vi "Start Drive Ref.vi"(8 "error in":errorcluster, 9 "Variant":variant, 10 "cluster":T2 {"Gyro"."Sample Rate" min=0.25 max=100.0 step=0.25}, 11 "VI in":T1) -> (0 "error out":errorcluster)   [LabVIEW 2016, in "Drive System.lvlib"]
uses:
  Drive System.lvlib
  <vilib>/Rock Robotics/WPI/Solenoid/WPI_SolenoidChannel.ctl
  <vilib>/Rock Robotics/WPI/Solenoid/WPI_SolenoidDevRef.ctl
  Varient Cmd Types/Lock Command.ctl
  <vilib>/Rock Robotics/SystemInterfaces/spilib/spi_bus.ctl
  <vilib>/Rock Robotics/SystemInterfaces/AI/FPGA_AIChannel.ctl
  <vilib>/Rock Robotics/WPI/Gyro/WPI_GyroDevRef.ctl
  <vilib>/Rock Robotics/SystemInterfaces/Encoder/FPGA_EncoderIdx.ctl
  <vilib>/Rock Robotics/WPI/Encoder/WPI_EncoderType.ctl
  <vilib>/Rock Robotics/SystemInterfaces/Counter/FPGA_CounterCtrSystemIndex.ctl
  <vilib>/Rock Robotics/WPI/Encoder/WPI_EncoderDevRef.ctl
  <vilib>/Rock Robotics/SystemInterfaces/DIO/FPGA_DIOPWMChannel.ctl
  <vilib>/Rock Robotics/WPI/PWM/WPI_PWMDeadband.ctl
  <vilib>/Rock Robotics/WPI/MotorControl/WPI_MotorControlType.ctl
  <vilib>/Rock Robotics/WPI/MotorControl/WPI_MotorControlDeviceRef.ctl
  <vilib>/Rock Robotics/WPI/RobotDrive/WPI_RobotDriveDevRef.ctl
  DriveCmdList.ctl
  DriveCmd.ctl
  DriveMainType.ctl
  Drive Refs/Drive Ref Type.ctl
panel:
  # "Analog"
  # "XRS"
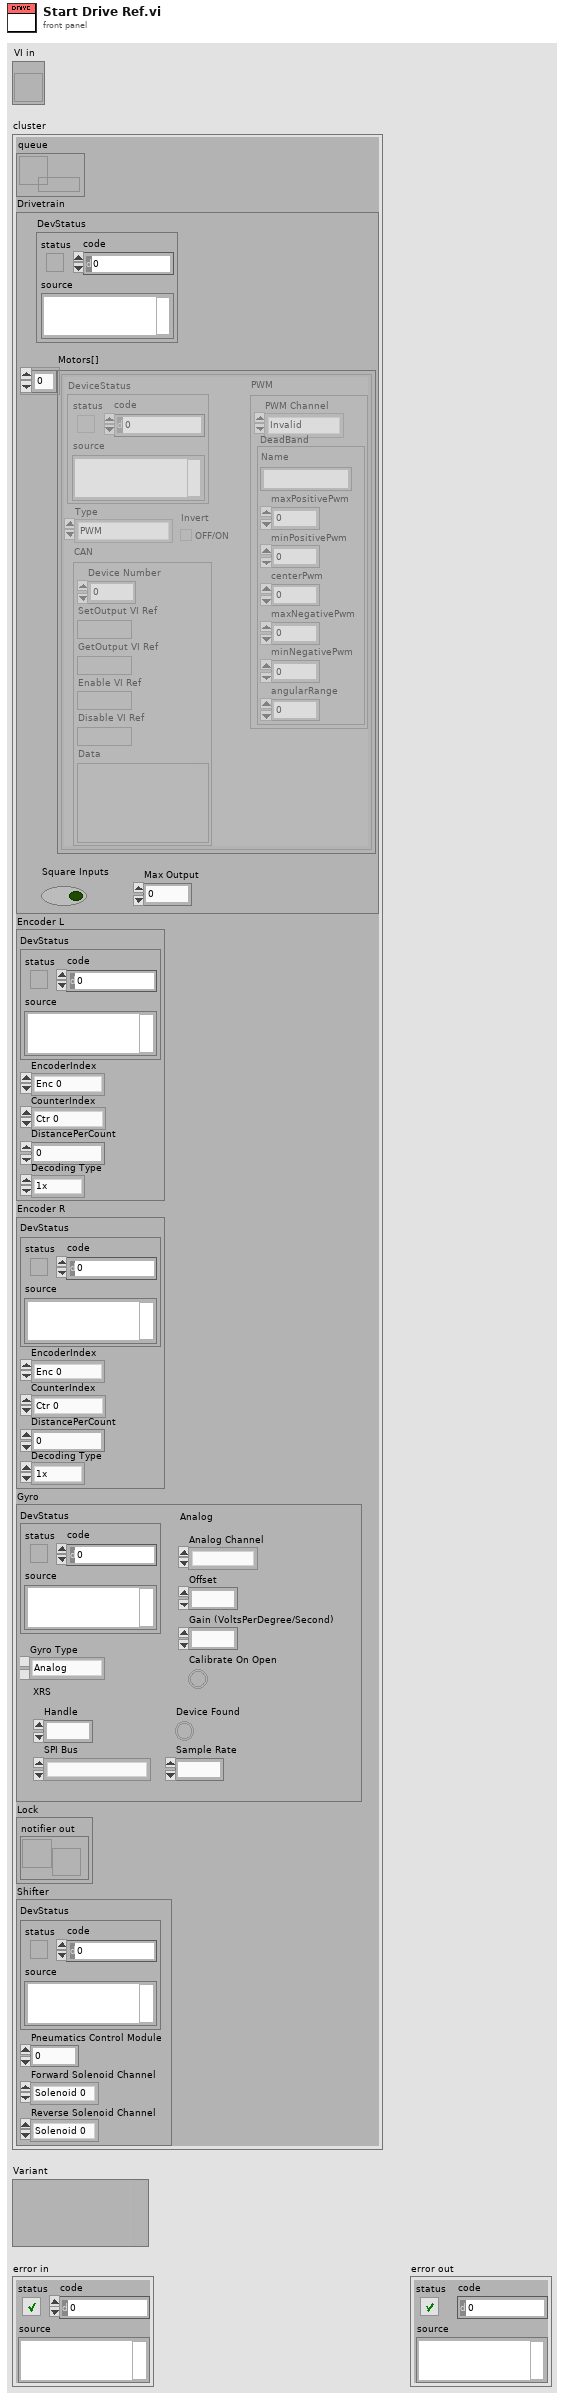
[diagram p1: front panel]
types:
  T1 = typedef "Drive System.lvlib/Drive Ref Type.ctl" = refnum<vi>
  T2 = typedef "Drive System.lvlib/DriveMainType.ctl" = cluster{"queue":refnum<queue>, "Drivetrain":T3, "Encoder L":T8, "Encoder R":T8, "Gyro":T12, "Lock":T15, "Shifter":T16}
  T3 = typedef "WPI_RobotDriveDevRef.ctl" = cluster{"DevStatus":errorcluster, "Motors[]":T4[], "Square Inputs":bool, "Max Output":dbl}
  T4 = typedef "WPI_MotorControlDeviceRef.ctl" = cluster{"DeviceStatus":errorcluster, "Type":T5, "PWM":cluster{"PWM Channel":T6, "DeadBand":T7}, "CAN":cluster{"Device Number":u8, "SetOutput VI Ref":variant, "GetOutput VI Ref":variant, "Enable VI Ref":variant, "Disable VI Ref":variant, "Data":variant}, "Invert":bool}
  T5 = typedef "WPI_MotorControlType.ctl" = enum16{"PWM", "CAN"}
  T6 = typedef "FPGA_DIOPWMChannel.ctl" = enum8{"PWM 0", "PWM 1", "PWM 2", "PWM 3", "PWM 4", "PWM 5", "PWM 6", "PWM 7", "PWM 8", "PWM 9", "PWM MXP 0", "PWM MXP 1", "PWM MXP 2", "PWM MXP 3", "PWM MXP 4", "PWM MXP 5", "PWM MXP 6", "PWM MXP 7", "PWM MXP 8", "PWM MXP 9", "Invalid"}
  T7 = typedef "WPI_PWMDeadband.ctl" = cluster{"Name":string, "maxPositivePwm":i32, "minPositivePwm":i32, "centerPwm":i32, "maxNegativePwm":i32, "minNegativePwm":i32, "angularRange":u16}
  T8 = typedef "WPI_EncoderDevRef.ctl" = cluster{"DevStatus":errorcluster, "EncoderIndex":T9, "CounterIndex":T10, "DistancePerCount":dbl, "Decoding Type":T11}
  T9 = typedef "FPGA_EncoderIdx.ctl" = enum8{"Enc 0", "Enc 1", "Enc 2", "Enc 3", "Enc 4", "Enc 5", "Enc 6", "Enc 7", "Invalid"}
  T10 = typedef "FPGA_CounterCtrSystemIndex.ctl" = enum8{"Ctr 0", "Ctr 1", "Ctr 2", "Ctr 3", "Ctr 4", "Ctr 5", "Ctr 6", "Ctr 7", "Invalid"}
  T11 = typedef "WPI_EncoderType.ctl" = enum16{"1x", "2x", "4x"}
  T12 = typedef "WPI_GyroDevRef.ctl" = cluster{"DevStatus":errorcluster, "Analog Channel":T13, "Offset":dbl, "Gain (VoltsPerDegree/Second)":dbl, "Gyro Type":enum16{"Analog", "XRS450"}, "Handle":i32, "SPI Bus":T14, "Device Found":bool, "Sample Rate":dbl, "Calibrate On Open":bool}
  T13 = typedef "FPGA_AIChannel.ctl" = enum8{"AI 0", "AI 1", "AI 2", "AI 3", "AI MXP 0", "AI MXP 1", "AI MXP 2", "AI MXP 3", "Invalid"}
  T14 = typedef "spi_bus.ctl" = enum16{"SPI On-Board, CS0", "SPI On-Board, CS1", "SPI On-Board, CS2", "SPI On-Board, CS3", "SPI MXP", "Invalid"}
  T15 = typedef "Drive System.lvlib/Lock Command.ctl" = cluster{"notifier out":refnum<notifier>}
  T16 = typedef "WPI_SolenoidDevRef.ctl" = cluster{"DevStatus":errorcluster, "Pneumatics Control Module":u8, "Forward Solenoid Channel":T17, "Reverse Solenoid Channel":T17}
  T17 = typedef "WPI_SolenoidChannel.ctl" = enum8{"Solenoid 0", "Solenoid 1", "Solenoid 2", "Solenoid 3", "Solenoid 4", "Solenoid 5", "Solenoid 6", "Solenoid 7", "Invalid"}
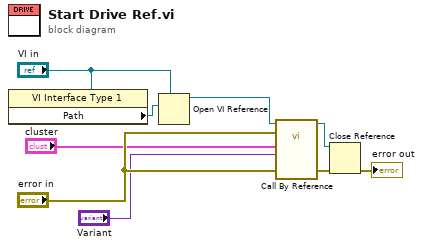
[diagram p0: block diagram]
diagram:
  n1 = property class="VI Interface Type 1"(reference="VI in") -> ("Path"=w3:path)  [unwired: 1 in, 2 out]
  n2 = Open VI Reference(type specifier VI Refnum (for type only)="VI in", vi path=w3) -> (vi reference=w2:T1)  [unwired: 4 in, 1 out]
  n3 = call-by-ref "?"(reference=w2, error in="error in", "error in"="error in", "data"="Variant", "DriveRef"="cluster") -> (reference out=w8:T1, "error out"=w6:errorcluster)  [unwired: 8 in, 1 out]
  n4 = Close Reference(reference=w8, error in (no error)=w6) -> (error out=→"error out":errorcluster)
